vi "Output Action.vi"(8 "error in (no error)":errorcluster, 9 "data":variant, 10 "type":string, 11 "Device in":refnum<class "Device.lvclass">) -> (0 "error out":errorcluster, 3 "Device out":refnum<class "Device.lvclass">)   [LabVIEW 2023, in "Device.lvlib" / "Device.lvclass"]
uses:
  Device.lvclass
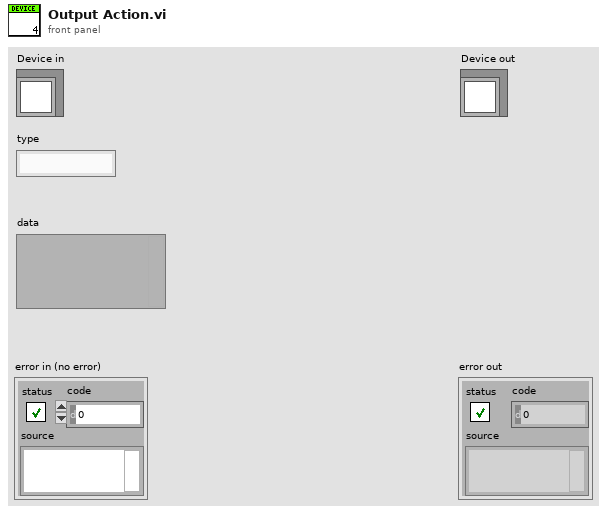
[diagram p1: front panel]
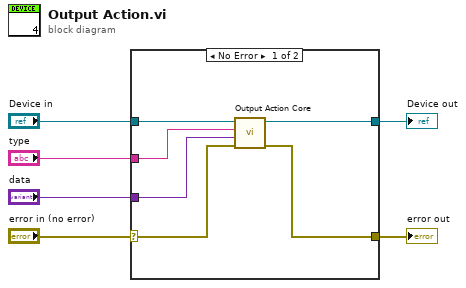
[diagram p0: block diagram]
diagram:
  n1 = case shown="No Error" "error in (no error)" {
    selector: "error in (no error)" -> [w10 w14]
    tunnel: [w9 w14] -> w5
    tunnel: [w11 w13] -> w3
    tunnel: "Device in" -> [w12 w13]
    tunnel: "type" -> [w8 _]
    tunnel: "data" -> [w7 _]
    frame No Error {
      n2 = call-dynamic "Output Action Core.vi"("error in (no error)"=w10, "data"=w7, "type"=w8, "Device in"=w12) -> ("error out"=w9:errorcluster, "Device out"=w11:refnum<class "Device.lvclass">)  [unwired: 6 in]
    }
    frame Error {
    }
  }
  "error out" <- w5
  "Device out" <- w3
